vi "Contour Arc Length.vi"(7 "Is Closed? (Default: True)":bool=TRUE, 8 "error in (no error)":errorcluster, 11 "Points in":T1[](array[typedef])) -> (0 "error out":errorcluster, 3 "Arc Length":dbl)   [LabVIEW 2020, in "shape.lvlib"]
doc: "Compute the Arc Length of a given Contour."
uses:
  shape.lvlib
  common/Image Point (Integer).ctl
  common/common.lvlib
  common/bin/gartoolkit_32-1.dll
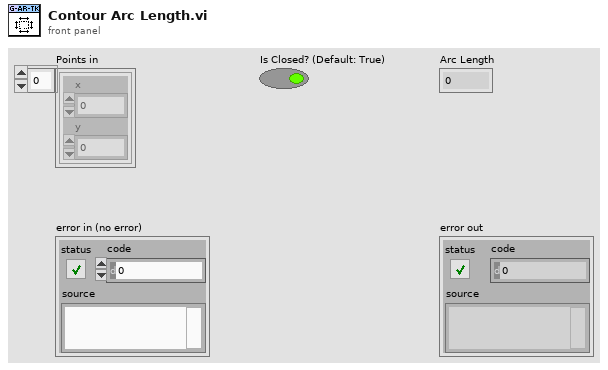
[diagram p1: front panel]
types:
  T1 = typedef "common.lvlib/Image Point (Integer).ctl" = cluster{"x":i32, "y":i32}
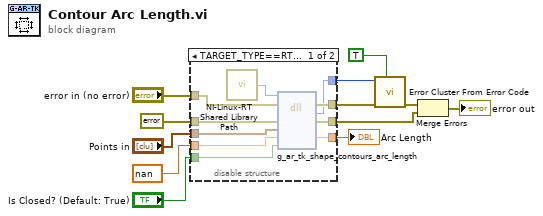
[diagram p0: block diagram]
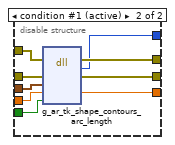
[diagram p2: hidden frame]
diagram:
  n1 = disable-structure shown="TARGET_TYPE==RT&&OS==Linux" {
    disable-tunnel: "error in (no error)" -> [w22 w31]
    disable-tunnel: errorcluster {"status"=FALSE, "code"=0, "source"=""} ("error constant") -> [w21 w30]
    disable-tunnel: "Points in" -> [w20 w29]
    disable-tunnel: nan ("arc_length") -> [w19 w28]
    disable-tunnel: "Is Closed? (Default: True)" -> [w18 w27]
    disable-tunnel: [w17 w26] -> w5
    disable-tunnel: [w16 w25] -> w4
    disable-tunnel: [w15 w24] -> w3
    disable-tunnel: [w14 w23] -> w2
    frame condition #0 {
      n2 = call "NI-Linux-RT Shared Library Path.vi"() -> ("Path"=w13:path)
      n3 = dll-call lib="?" fn="g_ar_tk_shape_contours_arc_length" ("g_ar_toolkit.*.*:g_ar_tk_image_draw_line")(path in=w13, error in=w22, "error_cluster"=w21, "points"=w20, "arc_length"=w19, "is_closed"=w18) -> (error out=w17:errorcluster, "MgErr"=w16:i32, "error_cluster"=w15:errorcluster, "arc_length"=w14:dbl)  [unwired: 3 in, 1 out]
    }
    frame condition #1 (active) {
      n4 = dll-call lib="C:/serenial/lib/g-augmented-reality-toolkit/LabVIEW/common/bin/gartoolkit_*-1.*" fn="g_ar_tk_shape_contours_arc_length" ("g_ar_toolkit.*.*:g_ar_tk_image_draw_line")(error in=w31, "error_cluster"=w30, "points"=w29, "arc_length"=w28, "is_closed"=w27) -> (error out=w26:errorcluster, "MgErr"=w25:i32, "error_cluster"=w24:errorcluster, "arc_length"=w23:dbl)  [unwired: 4 in, 1 out]
    }
  }
  "Arc Length" <- w2
  n5 = call <vilib>:"Error Cluster From Error Code.vi"("show call chain? (False)"=TRUE, "error in (no error)"=w5, "error code (0)"=w4) -> ("error out"=w11:errorcluster)  [unwired: 6 in]
  n6 = Merge Errors(w11, w3) -> (→"error out":errorcluster)
